vi "wcssph2xy.vi"(8 "lat":dbl format="%.6g", 9 "lon":dbl, 11 "Astrometry":T1 {"CRVAL" format="%.6g"; "CD" format="%_7g"}) -> (0 "Y":dbl, 1 "X":dbl)   [LabVIEW 2011]
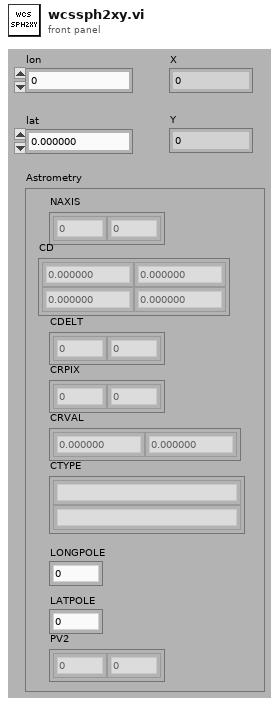
[diagram p1: front panel]
types:
  T1 = cluster{"NAXIS":dbl[], "CD":dbl[][], "CDELT":dbl[], "CRPIX":dbl[], "CTYPE":string[], "CRVAL":dbl[], "LONGPOLE":dbl, "LATPOLE":dbl, "PV2":dbl[]}
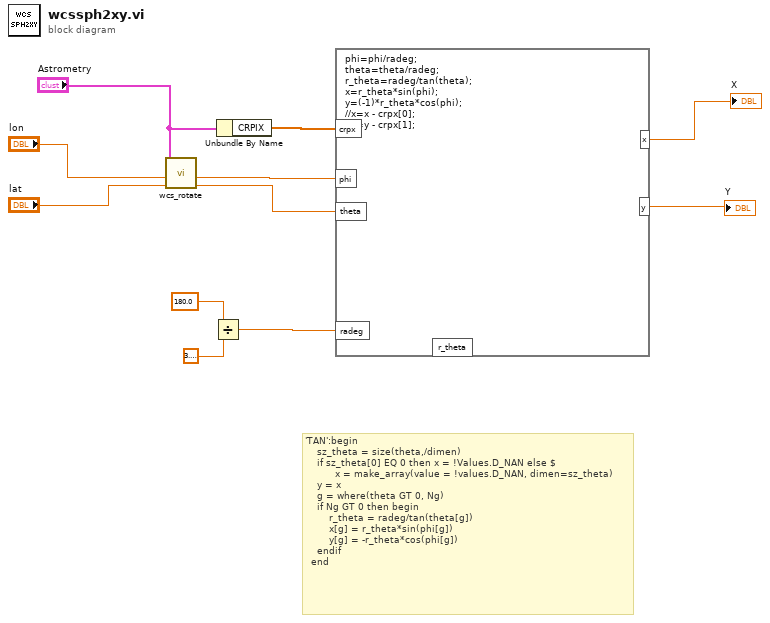
[diagram p0: block diagram]
diagram:
  # "'TAN':begin\n    sz_theta = size(theta,/dimen)\n    if sz_theta[0] EQ 0 then x = !Values.D_NAN else $\n          x = make_array(value = !values.D_NAN, dimen=sz_theta)\n    y = x\n    g = where(theta GT 0, Ng)\n    if Ng GT 0 then begin\n        r_theta = radeg/tan(theta[g])\n        x[g] = r_theta*sin(phi[g])\n        y[g] = -r_theta*cos(phi[g])\n    endif\n  end"
  n1 = call "wcs_rotate.vi"("latitude"="lat", "longitude"="lon", "Astrometry"="Astrometry") -> ("theta"=w8:dbl, "phi"=w9:dbl)  [unwired: 7 in]
  n2 = Divide(x=180.0, y=3.141592653589793) -> (x/y=w7:dbl)
  n3 = Unbundle By Name("Astrometry") -> ("CRPIX"=w1:dbl[])
  n4 = formula code="phi=phi/radeg;\ntheta=theta/radeg;\nr_theta=radeg/tan(theta);\nx=r_theta*sin(phi);\ny=(-1)*r_theta*cos(phi);\n//x=x - crpx[0];\n//y=y - crpx[1];"("phi"=w9, "theta"=w8, "radeg"=w7, "crpx"=w1) -> ("x"=→"X":dbl, "y"=→"Y":dbl)  [unwired: 1 out]
